vi "startUp.vi"(8 "error in (no error)":errorcluster, 10 "HardwareList out":refnum<class "HWConfiguration.lvclass">, 11 "BECHWCBasic in":refnum<class "BECHWCBasic.lvclass">) -> (0 "error out":errorcluster, 3 "BECHWCBasic out":refnum<class "BECHWCBasic.lvclass">)   [LabVIEW 2009, in "Hardware.lvlib" / "HWControllers.lvlib" / "BECHWCBasic.lvclass"]
doc: "Opens the devices ready for use."
uses:
  BECHWCBasic.lvclass
  HardwareConfiguration/HWConfiguration.lvclass
  BECHWCBasic.lvclass/BECHWCBasic.ctl
  Channels/Digital/DigitalOutput.lvclass
  Channels/VoltOutput/AnalogOutput.lvclass
  HWController.lvclass
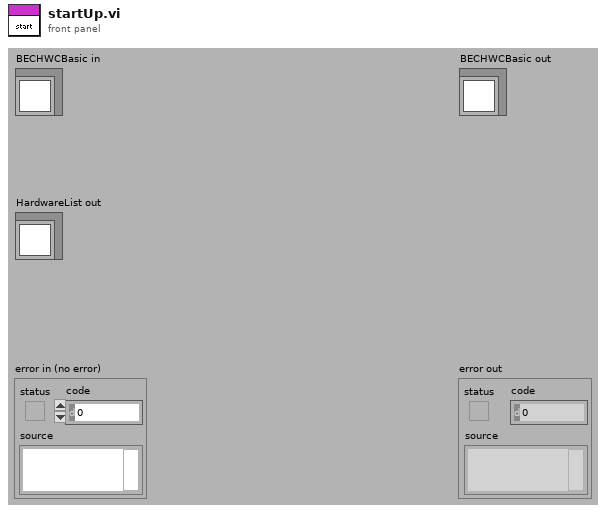
[diagram p1: front panel]
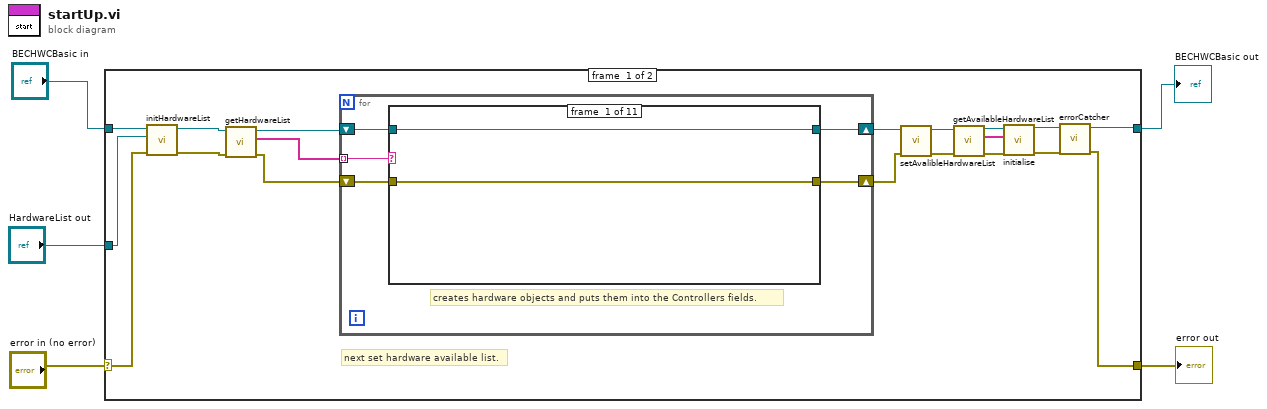
[diagram p0: block diagram]
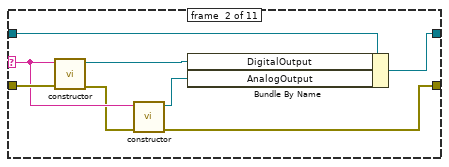
[diagram p2: hidden frame]
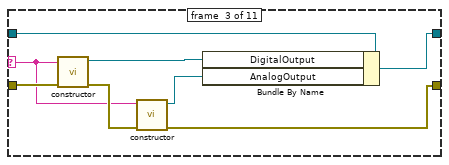
[diagram p3: hidden frame]
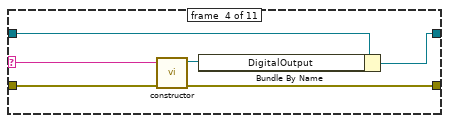
[diagram p4: hidden frame]
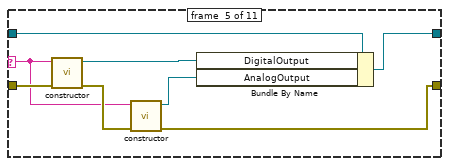
[diagram p5: hidden frame]
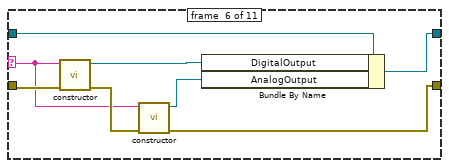
[diagram p6: hidden frame]
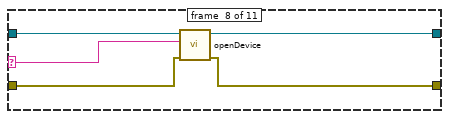
[diagram p8: hidden frame]
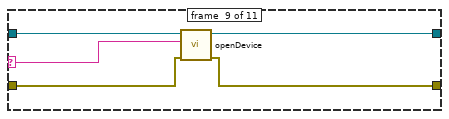
[diagram p9: hidden frame]
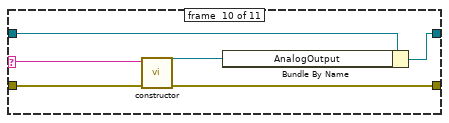
[diagram p10: hidden frame]
diagram:
  n1 = case shown="No Error" "error in (no error)" {
    selector: "error in (no error)" -> [w7 w90]
    tunnel: [w10 w90] -> w4
    tunnel: "BECHWCBasic in" -> [w8 w91]
    tunnel: [w9 w91] -> w2
    tunnel: "HardwareList out" -> [w6 _]
    frame #0 {
      # "next set hardware available list."
      n2 = call-dynamic "initHardwareList.vi"("error in (no error)"=w7, "HardwareList out"=w6, "BECHWCBasic in"=w8) -> ("error out"=w20:errorcluster, "BECHWCBasic out"=w22:refnum<class "BECHWCBasic.lvclass">)  [unwired: 7 in]
      n3 = call "getHardwareList.vi"("error in (no error)"=w20, "HWController.lvclass in"=w22) -> ("error out"=w19:errorcluster, "HardwareList"=w18:string[], "HWController.lvclass out"=w21:refnum<class "BECHWCBasic.lvclass">)  [unwired: 7 in]
      n4 = for {
        tunnel: w18 -> [w29] mode=indexing
        shift-right: [w27] -> w24
        shift-left: w21 -> [w28]
        shift-right: [w25] -> w23
        shift-left: w19 -> [w26]
        # "creates hardware objects and puts them into the Controllers fields."
        n5 = case shown="\"S1010\"" w29 {
          selector: w29 -> [_ w38 w40 w49 w57 w62 _ w72 w77 w87 _]
          tunnel: w28 -> [w31 w35 w43 w50 w55 w65 w71 w76 w81 w85 w89]
          tunnel: [w31 w32 w42 w51 w54 w64 w71 w75 w80 w84 w89] -> w27
          tunnel: w26 -> [w30 w39 w44 w48 w58 w66 w70 w74 w78 w86 w88]
          tunnel: [w30 w36 w41 w52 w56 w63 w70 w73 w79 w82 w88] -> w25
          frame #0 {
          }
          frame #1 {
            n6 = call "constructor.vi"("error in (no error)"=w39, "deviceName"=w38) -> ("error out"=w37:errorcluster, "DigitalOutput out"=w34:refnum<class "DigitalOutput.lvclass">)  [unwired: 8 in]
            n7 = call "constructor.vi"("error in (no error)"=w37, "deviceName"=w38) -> ("error out"=w36:errorcluster, "AnalogOutput out"=w33:refnum<class "AnalogOutput.lvclass">)  [unwired: 8 in]
            n8 = Bundle By Name(cluster=w35, "DigitalOutput"=w34, "AnalogOutput"=w33) -> (w32:refnum<class "BECHWCBasic.lvclass">)
          }
          frame #2 {
            n9 = call "constructor.vi"("error in (no error)"=w44, "deviceName"=w40) -> ("error out"=w47:errorcluster, "DigitalOutput out"=w46:refnum<class "DigitalOutput.lvclass">)  [unwired: 8 in]
            n10 = call "constructor.vi"("error in (no error)"=w47, "deviceName"=w40) -> ("error out"=w41:errorcluster, "AnalogOutput out"=w45:refnum<class "AnalogOutput.lvclass">)  [unwired: 8 in]
            n11 = Bundle By Name(cluster=w43, "DigitalOutput"=w46, "AnalogOutput"=w45) -> (w42:refnum<class "BECHWCBasic.lvclass">)
          }
          frame #3 {
            n12 = call "constructor.vi"("error in (no error)"=w48, "deviceName"=w49) -> ("error out"=w52:errorcluster, "DigitalOutput out"=w53:refnum<class "DigitalOutput.lvclass">)  [unwired: 8 in]
            n13 = Bundle By Name(cluster=w50, "DigitalOutput"=w53) -> (w51:refnum<class "BECHWCBasic.lvclass">)
          }
          frame #4 {
            n14 = call "constructor.vi"("error in (no error)"=w58, "deviceName"=w57) -> ("error out"=w61:errorcluster, "DigitalOutput out"=w60:refnum<class "DigitalOutput.lvclass">)  [unwired: 8 in]
            n15 = call "constructor.vi"("error in (no error)"=w61, "deviceName"=w57) -> ("error out"=w56:errorcluster, "AnalogOutput out"=w59:refnum<class "AnalogOutput.lvclass">)  [unwired: 8 in]
            n16 = Bundle By Name(cluster=w55, "DigitalOutput"=w60, "AnalogOutput"=w59) -> (w54:refnum<class "BECHWCBasic.lvclass">)
          }
          frame #5 {
            n17 = call "constructor.vi"("error in (no error)"=w66, "deviceName"=w62) -> ("error out"=w69:errorcluster, "DigitalOutput out"=w68:refnum<class "DigitalOutput.lvclass">)  [unwired: 8 in]
            n18 = call "constructor.vi"("error in (no error)"=w69, "deviceName"=w62) -> ("error out"=w63:errorcluster, "AnalogOutput out"=w67:refnum<class "AnalogOutput.lvclass">)  [unwired: 8 in]
            n19 = Bundle By Name(cluster=w65, "DigitalOutput"=w68, "AnalogOutput"=w67) -> (w64:refnum<class "BECHWCBasic.lvclass">)
          }
          frame #6 {
          }
          frame #7 {
            n20 = call "openDevice.vi"("error in (no error)"=w74, "deviceName"=w72, "BECHWCBasic in"=w76) -> ("error out"=w73:errorcluster, "BECHWCBasic out"=w75:refnum<class "BECHWCBasic.lvclass">)  [unwired: 7 in]
          }
          frame #8 {
            n21 = call "openDevice.vi"("error in (no error)"=w78, "deviceName"=w77, "BECHWCBasic in"=w81) -> ("error out"=w79:errorcluster, "BECHWCBasic out"=w80:refnum<class "BECHWCBasic.lvclass">)  [unwired: 7 in]
          }
          frame #9 {
            n22 = call "constructor.vi"("error in (no error)"=w86, "deviceName"=w87) -> ("error out"=w82:errorcluster, "AnalogOutput out"=w83:refnum<class "AnalogOutput.lvclass">)  [unwired: 8 in]
            n23 = Bundle By Name(cluster=w85, "AnalogOutput"=w83) -> (w84:refnum<class "BECHWCBasic.lvclass">)
          }
          frame #10 {
          }
        }
      }
      n24 = call "setAvalibleHardwareList.vi"("error in (no error)"=w23, "HWController in"=w24) -> ("error out"=w16:errorcluster, "HWController out"=w17:refnum<class "BECHWCBasic.lvclass">)  [unwired: 8 in]
      n25 = call "getAvailableHardwareList.vi"("error in (no error)"=w16, "HWController.lvclass in"=w17) -> ("error out"=w14:errorcluster, "AvailableHardwareList"=w13:string[], "HWController.lvclass out"=w15:refnum<class "BECHWCBasic.lvclass">)  [unwired: 7 in]
      n26 = call-dynamic "initialise.vi"("error in (no error)"=w14, "HWList"=w13, "BECHWCBasic in"=w15) -> ("error out"=w11:errorcluster, "BECHWCBasic out"=w12:refnum<class "BECHWCBasic.lvclass">)  [unwired: 7 in]
      n27 = call-dynamic "errorCatcher.vi"("error in (no error)"=w11, "HWController in"=w12) -> ("error out"=w10:errorcluster, "HWController out"=w9:refnum<class "BECHWCBasic.lvclass">)  [unwired: 8 in]
    }
    frame #1 {
    }
  }
  "error out" <- w4
  "BECHWCBasic out" <- w2
